vi "Parse Port (Tx-UDP-SAP).vi"(8 "error in":errorcluster, 11 "node in":refnum<k20>) -> (0 "error out":errorcluster, 3 "tx udp sap port out":T1={"PayloadID"="", "SubVlId"=1, "UdpSrcPort"=0, "UdpNumBufMessages"=0, "UdpMaxMessageSize"=128, "partitionID"=0, "domainID"=0, "sideID"=0, "locationID"=0, "interfaceID"=0, "Parameters"=[]} {"Parameters"."Parameter"."encoding" items=["BNR", "BCD", "Discrete"]})   [LabVIEW 2020, in "AIM ARINC 664 Import.lvlib"]
uses:
  AIM ARINC 664 Import.lvlib
  _typedefs/port_tx_udp_sap.ctl
  _typedefs/frame_parameter.ctl
  _typedefs/frame_parameter_definition.ctl
  Shared/Encoding (Arinc664).ctl
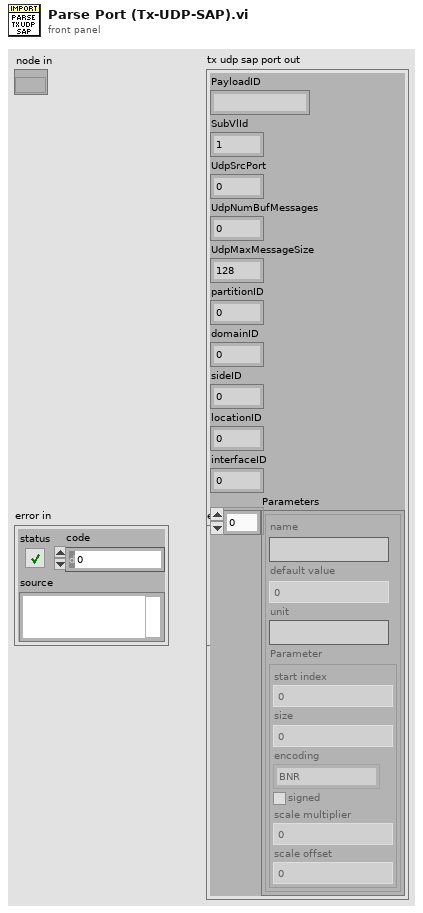
[diagram p1: front panel]
types:
  T1 = typedef "AIM ARINC 664 Import.lvlib/port_tx_udp_sap.ctl" = cluster{"PayloadID":string, "SubVlId":u8, "UdpSrcPort":u16, "UdpNumBufMessages":u32, "UdpMaxMessageSize":u32, "partitionID":u8, "domainID":u8, "sideID":u8, "locationID":u8, "interfaceID":u8, "Parameters":T2[]}
  T2 = typedef "AIM ARINC 664 Import.lvlib/frame_parameter.ctl" = cluster{"name":string, "default value":dbl, "unit":string, "Parameter":T3}
  T3 = typedef "AIM ARINC 664 Import.lvlib/frame_parameter_definition.ctl" = cluster{"start index":i32, "size":i32, "encoding":T4, "signed":bool, "scale multiplier":dbl, "scale offset":dbl}
  T4 = typedef "Encoding (Arinc664).ctl" = u16
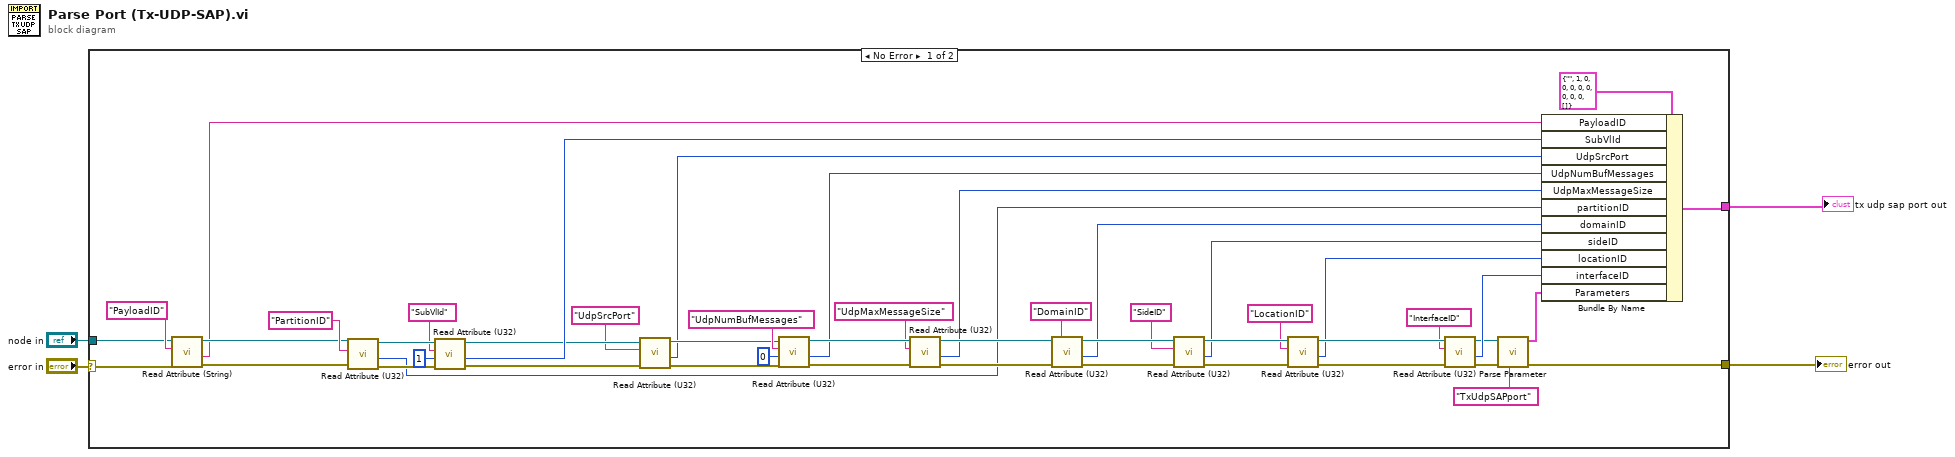
[diagram p0: block diagram]
diagram:
  n1 = case shown="No Error" "error in" {
    selector: "error in" -> [w8 w54]
    tunnel: "node in" -> [w9 _]
    tunnel: [w12 w54] -> w3
    tunnel: [w53 _] -> w1
    frame No Error {
      n2 = call "Read Attribute (String).vi"("error in"=w8, "Attribute Name"="PayloadID" ("Name"), "node in"=w9) -> ("error out"=w7:errorcluster, "value"=w5:string, "node out"=w6:refnum<k20>)  [unwired: 6 in]
      n3 = call "Read Attribute (U32).vi"("error in"=w7, "Attribute Name"="PartitionID" ("Tag Name"), "node in"=w6) -> ("error out"=w51:errorcluster, "value"=w18:u32, "node out"=w52:refnum<k20>)  [unwired: 6 in]
      n4 = call "Read Attribute (U32).vi"("error in"=w51, "default"=u32 1, "Attribute Name"="SubVlId" ("Tag Name"), "node in"=w52) -> ("error out"=w42:errorcluster, "value"=w48:u32, "node out"=w43:refnum<k20>)  [unwired: 5 in]
      n5 = call "Read Attribute (U32).vi"("error in"=w42, "Attribute Name"="UdpSrcPort" ("Tag Name"), "node in"=w43) -> ("error out"=w41:errorcluster, "value"=w38:u32, "node out"=w40:refnum<k20>)  [unwired: 6 in]
      n6 = call "Read Attribute (U32).vi"("error in"=w41, "default"=u32 0, "Attribute Name"="UdpNumBufMessages" ("Tag Name"), "node in"=w40) -> ("error out"=w47:errorcluster, "value"=w28:u32, "node out"=w46:refnum<k20>)  [unwired: 5 in]
      n7 = call "Read Attribute (U32).vi"("error in"=w47, "Attribute Name"="UdpMaxMessageSize" ("Tag Name"), "node in"=w46) -> ("error out"=w30:errorcluster, "value"=w27:u32, "node out"=w31:refnum<k20>)  [unwired: 6 in]
      n8 = call "Read Attribute (U32).vi"("error in"=w30, "Attribute Name"="DomainID" ("Tag Name"), "node in"=w31) -> ("error out"=w35:errorcluster, "value"=w22:u32, "node out"=w34:refnum<k20>)  [unwired: 6 in]
      n9 = call "Read Attribute (U32).vi"("error in"=w35, "Attribute Name"="SideID" ("Tag Name"), "node in"=w34) -> ("error out"=w36:errorcluster, "value"=w21:u32, "node out"=w37:refnum<k20>)  [unwired: 6 in]
      n10 = call "Read Attribute (U32).vi"("error in"=w36, "Attribute Name"="LocationID" ("Tag Name"), "node in"=w37) -> ("error out"=w32:errorcluster, "value"=w20:u32, "node out"=w33:refnum<k20>)  [unwired: 6 in]
      n11 = call "Read Attribute (U32).vi"("error in"=w32, "Attribute Name"="InterfaceID" ("Tag Name"), "node in"=w33) -> ("error out"=w15:errorcluster, "value"=w19:u32, "node out"=w14:refnum<k20>)  [unwired: 6 in]
      n12 = call "Parse Parameter.vi"("error text in"="TxUdpSAPport", "error in"=w15, "node in"=w14) -> ("error out"=w12:errorcluster, "parametesrs"=w13:T2[])  [unwired: 7 in]
      n13 = Bundle By Name(cluster=T1 {"PayloadID"="", "SubVlId"=1, "UdpSrcPort"=0, "UdpNumBufMessages"=0, "UdpMaxMessageSize"=0, "partitionID"=0, "domainID"=0, "sideID"=0, "locationID"=0, "interfaceID"=0, "Parameters"=[]} ("port_tx_udp_comm"), "PayloadID"=w5, "SubVlId"=w48, "UdpSrcPort"=w38, "UdpNumBufMessages"=w28, "UdpMaxMessageSize"=w27, "partitionID"=w18, "domainID"=w22, "sideID"=w21, "locationID"=w20, "interfaceID"=w19, "Parameters"=w13) -> (w53:T1)
    }
    frame Error {
    }
  }
  "error out" <- w3
  "tx udp sap port out" <- w1
